vi "Supply_ComplianceCheck.vi"(8 "error in (no error)":errorcluster, 11 "SupplyControl in":refnum<class "SupplyControl.lvclass">) -> (0 "error out":errorcluster, 1 "Status string":string, 2 "Compliance exceeded?":bool, 3 "SupplyControl out":refnum<class "SupplyControl.lvclass">)   [LabVIEW 2018, in "SupplyControl.lvclass"]
uses:
  SupplyControl.lvclass
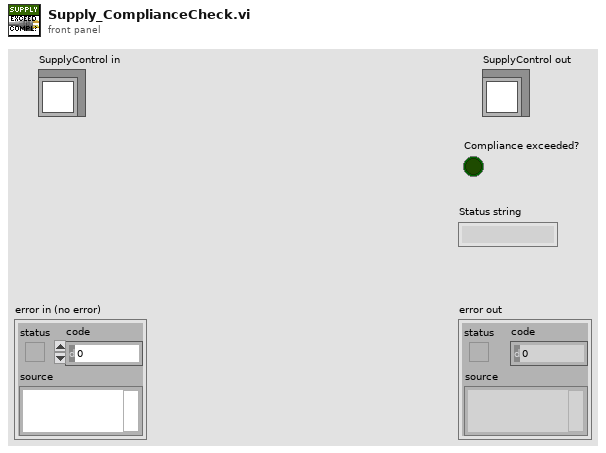
[diagram p1: front panel]
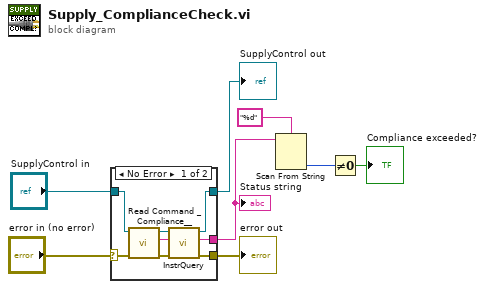
[diagram p0: block diagram]
diagram:
  n1 = case shown="No Error" "error in (no error)" {
    selector: "error in (no error)" -> [w9 w17]
    tunnel: [w16 w17] -> w8
    tunnel: [w15 w18] -> w7
    tunnel: "SupplyControl in" -> [w11 w18]
    tunnel: [w10 _] -> w4
    frame No Error {
      n2 = call-dynamic "Read Command _Compliance__.vi"("error in (no error)"=w9, "SupplyControl in"=w11) -> ("error out"=w14:errorcluster, "Command \"Compliance?\""=w13:string, "SupplyControl out"=w12:refnum<class "SupplyControl.lvclass">)  [unwired: 7 in]
      n3 = call-dynamic "InstrQuery.vi"("error in (no error)"=w14, "Command string"=w13, "InstControl in"=w12) -> ("error out"=w16:errorcluster, "Instrument response"=w10:string, "InstControl out"=w15:refnum<class "SupplyControl.lvclass">)  [unwired: 6 in]
    }
    frame Error {
    }
  }
  "SupplyControl out" <- w7
  "error out" <- w8
  "Status string" <- w4
  n4 = Scan From String(format string="%d", input string=w4) -> (output 1=w3:i32)  [unwired: 3 in, 3 out]
  n5 = Not Equal To 0?(x=w3) -> (x != 0?=→"Compliance exceeded?":bool)
